vi "std2fwhm.vi"(1 "std. dev.":dbl) -> (0 "FWHM":dbl)   [LabVIEW 2020]
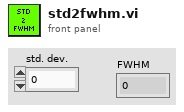
[diagram p1: front panel]
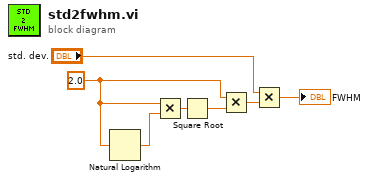
[diagram p0: block diagram]
diagram:
  w4 = 2.0
  n1 = Natural Logarithm(1:w4) -> (0:w6:dbl)
  n2 = Multiply(x=w4, y=w6) -> (x*y=w7:dbl)
  n3 = Square Root(x=w7) -> (sqrt(x)=w5:dbl)
  n4 = Multiply(x=w4, y=w5) -> (x*y=w3:dbl)
  n5 = Multiply(x="std. dev.", y=w3) -> (x*y=→"FWHM":dbl)
